vi "Write Name.vi"(8 "error in (no error)":errorcluster, 10 "Name":string, 11 "abs_Node in":refnum<class "abs_Node.lvclass">) -> (0 "error out":errorcluster, 3 "abs_Node out":refnum<class "abs_Node.lvclass">)   [LabVIEW 2021, in "BT.lvlib" / "abs_Node.lvclass"]
uses:
  abs_Node.lvclass
  abs_Node.lvclass/abs_Node.ctl
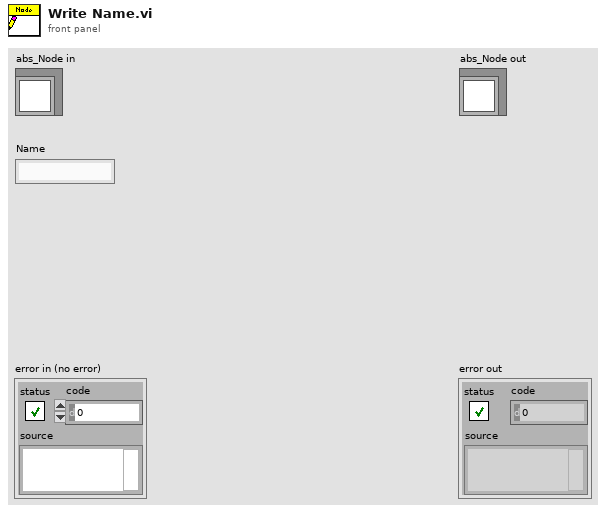
[diagram p1: front panel]
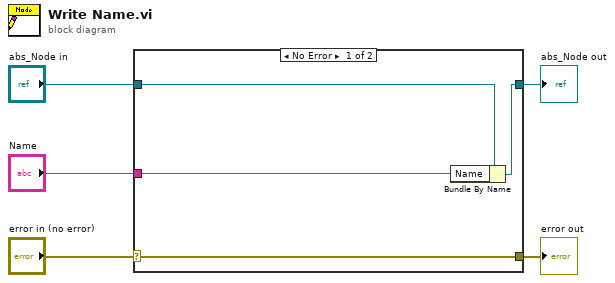
[diagram p0: block diagram]
diagram:
  n1 = case shown="No Error" "error in (no error)" {
    selector: "error in (no error)" -> [w9 w10]
    tunnel: [w9 w10] -> w4
    tunnel: [w7 w11] -> w2
    tunnel: "abs_Node in" -> [w8 w11]
    tunnel: "Name" -> [w6 _]
    frame No Error {
      n2 = Bundle By Name(cluster=w8, "Name"=w6) -> (w7:refnum<class "abs_Node.lvclass">)
    }
    frame Error {
    }
  }
  "error out" <- w4
  "abs_Node out" <- w2
